vi "Processing_Method.vi"(6 "Processin Mode":T1=enum."Drop by Threshold", 9 "FilterParams":variant, 10 "Original Data":dbl[](array[numeric])) -> (2 "Output":dbl[](array[numeric]))   [LabVIEW 2013]
uses:
  ControlDef/ProcessingMode.ctl
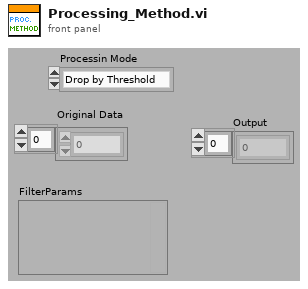
[diagram p1: front panel]
types:
  T1 = typedef "ProcessingMode.ctl" = enum16{"None", "Drop by Threshold", "TDC Simulate", "SetFilter"}
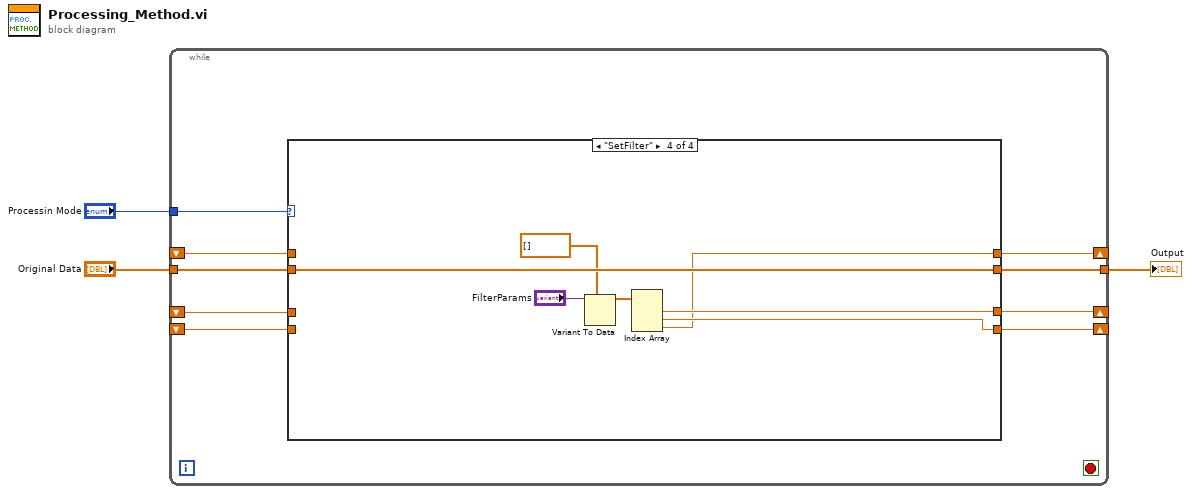
[diagram p0: block diagram]
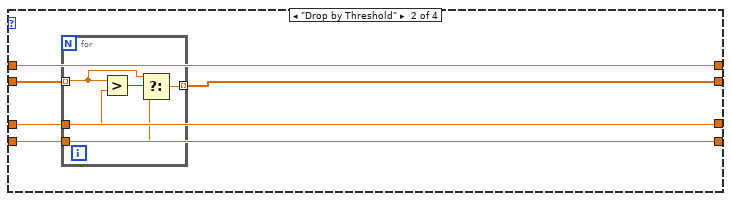
[diagram p3: hidden frame]
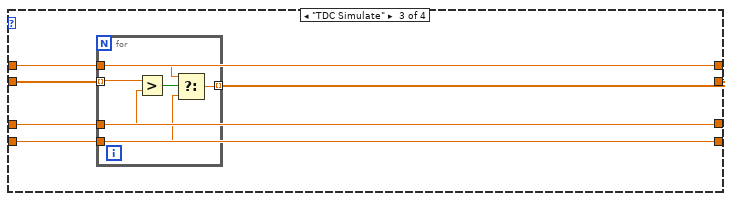
[diagram p4: hidden frame]
diagram:
  n1 = while {
    tunnel: [w10] -> w3
    tunnel: "Original Data" -> [w9]
    tunnel: "Processin Mode" -> [w8]
    shift-right: [w6] -> _
    shift-left: _ -> [w12]
    shift-right: [w4] -> _
    shift-left: _ -> [w7]
    shift-right: [w5] -> _
    shift-left: _ -> [w11]
    stop <- _ stop-if-true
    n2 = case shown="\"SetFilter\"" w8 {
      tunnel: w12 -> [w14 w21 w30 _]
      tunnel: w11 -> [w13 w20 w31 _]
      tunnel: [w16 w19 w28 w44] -> w10
      tunnel: w9 -> [w16 w18 w29 w44]
      tunnel: w7 -> [w15 w17 w27 _]
      tunnel: [w14 w21 w30 w41] -> w6
      tunnel: [w13 w20 w31 w40] -> w5
      tunnel: [w15 w17 w27 w39] -> w4
      frame "None", Default {
      }
      frame "Drop by Threshold" {
        n3 = for {
          tunnel: w18 -> [w25] mode=indexing
          tunnel: [w24] -> w19 mode=indexing
          tunnel: w20 -> [w23]
          tunnel: w21 -> [w22]
          n4 = Greater?(x=w25, y=w22) -> (0:w26:bool)
          n5 = Select(t=w25, s=w26, f=w23) -> (s? t:f=w24:dbl)
        }
      }
      frame "TDC Simulate" {
        n6 = for {
          tunnel: w29 -> [w36] mode=indexing
          tunnel: [w35] -> w28 mode=indexing
          tunnel: w31 -> [w34]
          tunnel: w30 -> [w33]
          tunnel: w27 -> [w32]
          n7 = Greater?(x=w36, y=w33) -> (0:w37:bool)
          n8 = Select(t=w32, s=w37, f=w34) -> (s? t:f=w35:dbl)
        }
      }
      frame "SetFilter" {
        n9 = Variant To Data(type=dbl[] [], Variant="FilterParams") -> (data=w42:dbl[])  [unwired: 1 in, 1 out]
        n10 = Index Array(array=w42) -> (element #1=w41:dbl, element #2=w40:dbl, element #3=w39:dbl)  [unwired: 3 in]
      }
    }
  }
  "Output" <- w3
